vi "Read Increment.vi"(8 "error in (no error)":errorcluster, 11 "Counter in":refnum<class "Counter.lvclass">) -> (0 "error out":errorcluster, 2 "Increment":i32, 3 "Counter out":refnum<class "Counter.lvclass">)   [LabVIEW 2015, in "Counter.lvclass"]
uses:
  Counter.lvclass
  Counter.lvclass/Counter.ctl
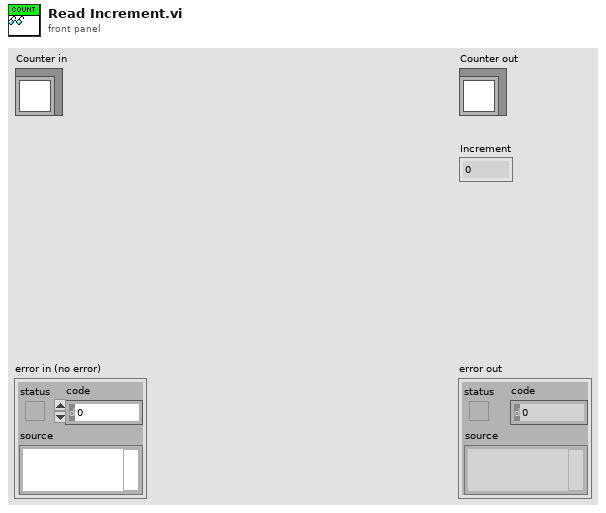
[diagram p1: front panel]
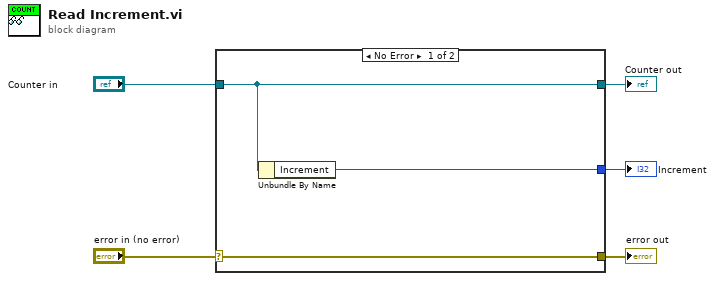
[diagram p0: block diagram]
diagram:
  n1 = case shown="No Error" "error in (no error)" {
    selector: "error in (no error)" -> [w8 w9]
    tunnel: [w8 w9] -> w4
    tunnel: [w7 w10] -> w2
    tunnel: "Counter in" -> [w7 w10]
    tunnel: [w6 _] -> w1
    frame No Error {
      n2 = Unbundle By Name(w7) -> ("Increment"=w6:i32)
    }
    frame Error {
    }
  }
  "error out" <- w4
  "Counter out" <- w2
  "Increment" <- w1
